vi "Dummy VI 3.vi"(7 "Numeric in":i32, 11 "String in":string) -> (3 "String out":string, 5 "Numeric out":i32)   [LabVIEW 2020]
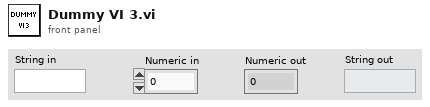
[diagram p1: front panel]
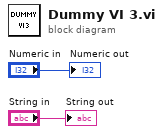
[diagram p0: block diagram]
diagram:
  "Numeric out" <- "Numeric in"
  "String out" <- "String in"
